vi "Autosampler Set Valve Pos.vi"(7 "Correlation ID":u32, 8 "error in (no error)":errorcluster, 10 "Valve Pos":u16, 11 "Application in":refnum<class "Application.lvclass">) -> (0 "error out":errorcluster, 3 "Application out":refnum<class "Application.lvclass">)   [LabVIEW 2023, in "Application.lvlib" / "Application.lvclass"]
uses:
  Application.lvclass
  Application.lvclass/Application.ctl
  Hardware/Device Messages/Save CorrID Msg/Save CorrID Msg.lvclass/Save CorrID Msg.ctl
  <vilib>/ActorFramework/Message Enqueuer/Message Enqueuer.lvclass/Message Enqueuer.ctl
  Hardware/Autosampler Messages/Set Valve Position Msg/Set Valve Position Msg.lvclass/Set Valve Position Msg.ctl
  <vilib>/ActorFramework/Message Enqueuer/Enqueue.vi
  Hardware/Device Messages/Save CorrID Msg/Save CorrID Msg.lvclass
  Hardware/Autosampler Messages/Set Valve Position Msg/Set Valve Position Msg.lvclass
  <vilib>/ActorFramework/Message Priority Queue/Priority Enqueue.vi
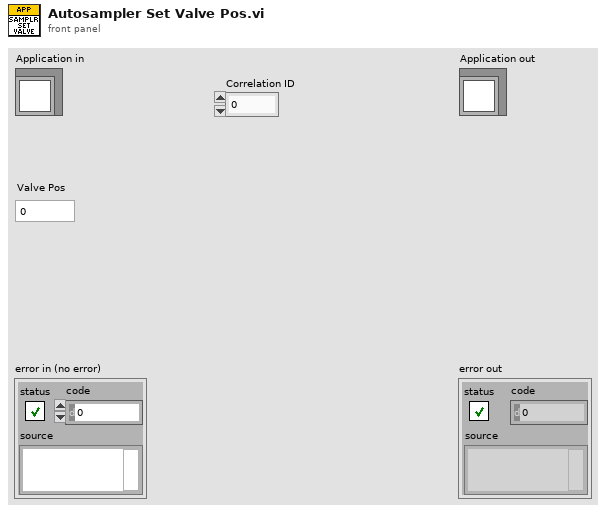
[diagram p1: front panel]
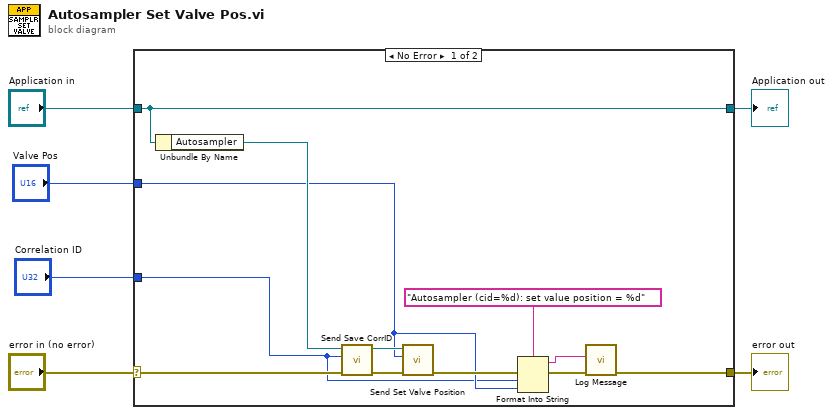
[diagram p0: block diagram]
diagram:
  n1 = case shown="No Error" "error in (no error)" {
    selector: "error in (no error)" -> [w12 w20]
    tunnel: [w14 w20] -> w5
    tunnel: [w18 w19] -> w3
    tunnel: "Application in" -> [w18 w19]
    tunnel: "Valve Pos" -> [w8 _]
    tunnel: "Correlation ID" -> [w7 _]
    frame No Error {
      n2 = Unbundle By Name(w18) -> ("Autosampler"=w10:refnum<class "Message Enqueuer.lvclass">)
      n3 = call "Send Save CorrID.vi"("error in (no error)"=w12, "Correlation ID"=w7, "Message Enqueuer"=w10) -> ("error out"=w11:errorcluster, "Message Enqueuer out"=w9:refnum<class "Message Enqueuer.lvclass">)  [unwired: 7 in]
      n4 = call "Send Set Valve Position.vi"("error in (no error)"=w11, "Valve Pos"=w8, "Message Enqueuer"=w9) -> ("error out"=w15:errorcluster)  [unwired: 7 in, 1 out]
      n5 = Format Into String(format string="Autosampler (cid=%d): set value position = %d", error in=w15, w7, w8) -> (resulting string=w17:string, error out=w16:errorcluster)  [unwired: 1 in]
      n6 = call "Log Message.vi"("error constant"=w16, "input"=w17) -> ("error constant 2"=w14:errorcluster)  [unwired: 8 in, 1 out]
    }
    frame Error {
    }
  }
  "error out" <- w5
  "Application out" <- w3
